vi "Kalman Filter.vi"   [LabVIEW 2014, in "Observer Library.lvlib" / "Kalman Filter.lvclass"]
uses:
  Kalman Filter.lvclass
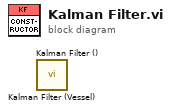
[diagram p0: block diagram]
diagram:
  n1 = call "Kalman Filter (Vessel).vi"() -> ()  [unwired: 11 in, 1 out]
  n2 = call "Kalman Filter ().vi"() -> ()  [unwired: 11 in, 1 out]
